vi "SPI Flash Read ID.vi"(10 "SPIIndex":i32, 11 "DevIndex":i32) -> (2 "function return":i32, 3 "pID":u8[](array[numeric]))   [LabVIEW 2010, in "usb2spi.lvlib"]
doc: "int WINAPI SPI_FlashReadID(int DevIndex,int SPIIndex,unsigned char *pID);"
uses:
  usb2spi.lvlib
  USB2XXX.dll
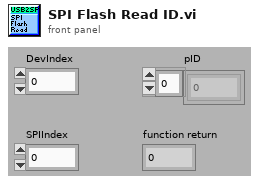
[diagram p1: front panel]
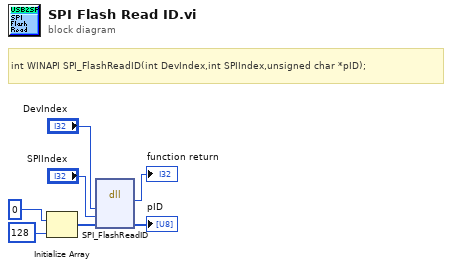
[diagram p0: block diagram]
diagram:
  # "int WINAPI SPI_FlashReadID(int DevIndex,int SPIIndex,unsigned char *pID);"
  n1 = Initialize Array(u8 0 ("element"), 128 ("dimension size")) -> (w4:u8[])
  n2 = dll-call lib="G:/OtherWork/USB2XXX_Example/trunk/Labview/PublicFiles/usb2spi/USB2XXX.*" fn="SPI_FlashReadID"("DevIndex"="DevIndex", "SPIIndex"="SPIIndex", "pID"=w4) -> (→"function return":i32, "pID"=→"pID":u8[])  [unwired: 5 in, 2 out]
